vi "Get SMO Public API.vi"(8 "error in (no error)":errorcluster, 11 "Instrument in":refnum<class "Instrument.lvclass">) -> (0 "error out":errorcluster, 2 "Commands":string[](array[string]), 3 "Instrument out":refnum<class "Instrument.lvclass">)   [LabVIEW 2019, in "Instrument.lvlib" / "Instrument.lvclass"]
doc: "Override this VI to return a list of commands supported by your Instrument"
uses:
  Instrument.lvclass
  Typedefs/Instrument.Commands--Enum.ctl
  a3a974a0-f424-49ae-9768-f4b353ce505d.vi
  <vilib>/Utility/Data Type/Get Numeric Information.vi
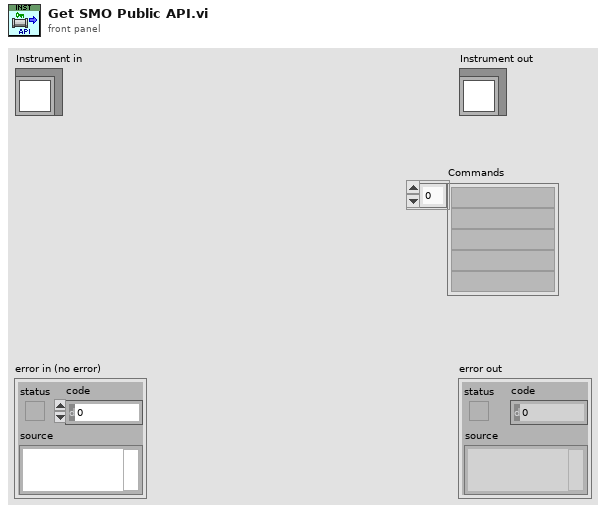
[diagram p1: front panel]
types:
  T1 = typedef "Instrument.lvlib/Instrument.lvclass/Instrument.Commands--Enum.ctl" = enum16{"ACK", "HELP", "setConfiguration", "setLogData", "getAll", "getAllData"}
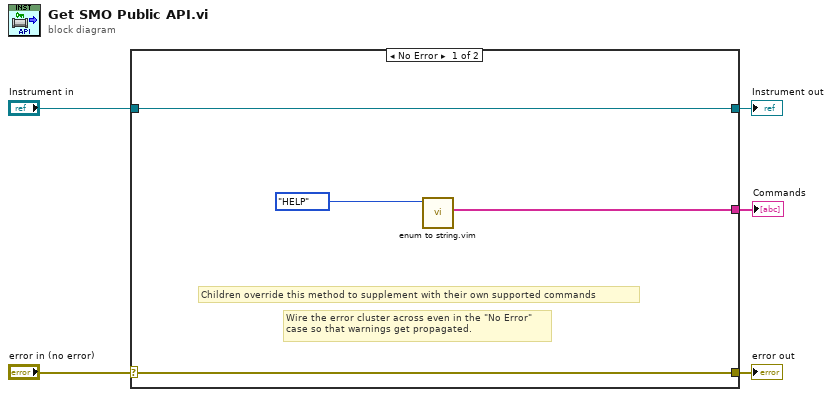
[diagram p0: block diagram]
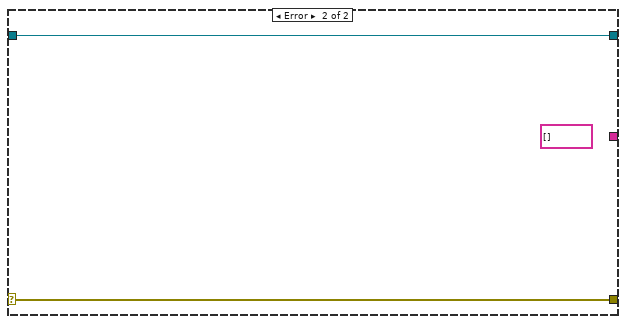
[diagram p2: hidden frame]
diagram:
  n1 = case shown="No Error" "error in (no error)" {
    selector: "error in (no error)" -> [w8 w11]
    tunnel: [w8 w11] -> w4
    tunnel: [w9 w10] -> w2
    tunnel: "Instrument in" -> [w9 w10]
    tunnel: [w6 _] -> w1
    frame No Error {
      # "Children override this method to supplement with their own supported commands"
      # "Wire the error cluster across even in the \"No Error\"\ncase so that warnings get propagated."
      n2 = call "enum to string.vim"("enum in"=Instrument.Commands--Enum."HELP" ("Commands")) -> ("strings out"=w6:string[])  [unwired: 9 in, 1 out]
    }
    frame Error {
      (unwired) string[] [] ("Array")
    }
  }
  "error out" <- w4
  "Instrument out" <- w2
  "Commands" <- w1
